vi "Check Dependencies with Preview.vi"(8 "error in (no error)":errorcluster, 11 "Builder in":refnum<class "Builder.lvclass">) -> (0 "error out":errorcluster, 3 "Builder out":refnum<class "Builder.lvclass">)   [LabVIEW 2019, in "Builder.lvclass"]
uses:
  Builder.lvclass
  Builder.lvclass/Builder.ctl
  <vilib>/Utility/lvfile.llb/LVFileType.ctl
  <vilib>/AppBuilder/AB_API/PPL/NI_AB_API_PPL.lvclass
  <vilib>/Utility/lvfile.llb/NI_FileType.lvlib
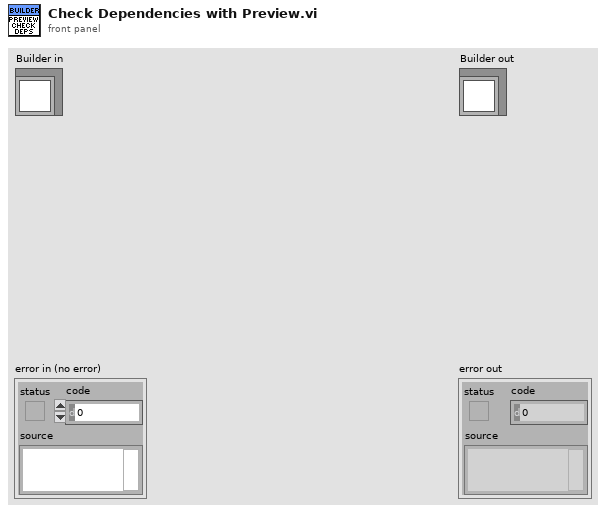
[diagram p1: front panel]
types:
  T1 = typedef "NI_FileType.lvlib/LVFileType.ctl" = enum32{"Invalid file", "Unknown type", "Instrument", "Control", "Polymorphic VI", "Project", "Library", "LVClass", "XControl", "XNode", "Shared library", ".NET assembly", "ActiveX interface", "CIN", "Run-time menu", "Palette menu", "Help file", "LLB", "XNode Edit Dependency", "Class Private Data Control", "Statechart", "MathScript .m file", "Ladder Diagram", "LVLibp", "XNode Build Dependency"}
  T2 = typedef "AB_Dependency.ctl" = cluster{"path":path, "delimited name":string, "type":T1}
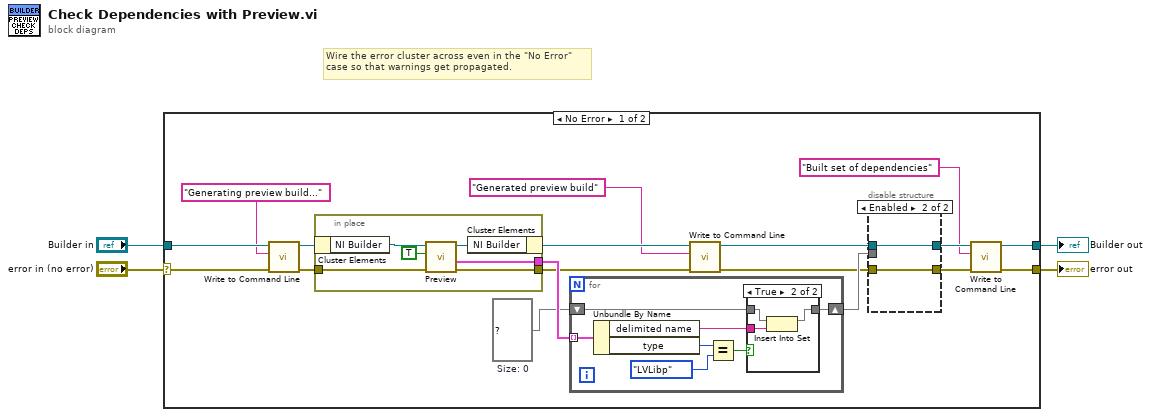
[diagram p0: block diagram]
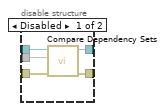
[diagram p2: hidden frame]
diagram:
  # "Wire the error cluster across even in the \"No Error\"\ncase so that warnings get propagated."
  n1 = case shown="No Error" "error in (no error)" {
    selector: "error in (no error)" -> [w22 w48]
    tunnel: [w10 w48] -> w3
    tunnel: [w8 w47] -> w1
    tunnel: "Builder in" -> [w15 w47]
    frame No Error {
      w20 = set{string} {}  # Size: 0
      n2 = call "Write to Command Line.vi"("error in (no error)"=w22, "Message"="Generating preview build...", "Builder in"=w15) -> ("error out"=w16:errorcluster, "Builder out"=w14:refnum<class "Builder.lvclass">)  [unwired: 7 in]
      n3 = in-place {
        in-place-border: w16 -> [w43]
        in-place-border: [w42] -> w18
        in-place-border: [w41] -> w21
        n4 = in-place-cluster #1(w14) -> ("NI Builder"=w46:refnum<class "NI_AB_API_PPL.lvclass">)
        n5 = call-dynamic "Preview.vi"("error in (no error)"=w43, "collect dependencies? (F)"=TRUE, "PPL in"=w46) -> ("error out"=w42:errorcluster, "Dependencies"=w41:T2[], "PPL out"=w45:refnum<class "NI_AB_API_PPL.lvclass">)  [unwired: 5 in, 1 out]
        n6 = in-place-cluster #1("NI Builder"=w45) -> (w12:refnum<class "Builder.lvclass">)
      }
      n7 = for {
        tunnel: w21 -> [w36] mode=indexing
        shift-right: [w31] -> w19
        shift-left: w20 -> [w30]
        n8 = Unbundle By Name(w36) -> ("delimited name"=w33:string, "type"=w35:T1)
        n9 = Equal?(x=w35, y=LVFileType."LVLibp") -> (x = y?=w32:bool)
        n10 = case shown="True" w32 {
          tunnel: w33 -> [_ w40]
          tunnel: [w37 w39] -> w31
          tunnel: w30 -> [w37 w38]
          frame False {
          }
          frame True {
            n11 = Insert Into Set(10:w40, 11:w38) -> (3:w39:set{string})  [unwired: 1 out]
          }
        }
      }
      n12 = call "Write to Command Line.vi"("error in (no error)"=w18, "Message"="Generated preview build", "Builder in"=w12) -> ("error out"=w13:errorcluster, "Builder out"=w11:refnum<class "Builder.lvclass">)  [unwired: 7 in]
      n13 = disable-structure shown="Enabled" {
        disable-tunnel: w19 -> [w27 _]
        disable-tunnel: w13 -> [w26 w28]
        disable-tunnel: [w25 w28] -> w17
        disable-tunnel: w11 -> [w24 w29]
        disable-tunnel: [w23 w29] -> w9
        frame Disabled {
          n14 = call "Compare Dependency Sets.vi"("error in (no error)"=w26, "Scanned"=w27, "Builder in"=w24) -> ("error out"=w25:errorcluster, "Builder out"=w23:refnum<class "Builder.lvclass">)  [unwired: 7 in]
        }
        frame Enabled {
        }
      }
      n15 = call "Write to Command Line.vi"("error in (no error)"=w17, "Message"="Built set of dependencies", "Builder in"=w9) -> ("error out"=w10:errorcluster, "Builder out"=w8:refnum<class "Builder.lvclass">)  [unwired: 7 in]
    }
    frame Error {
    }
  }
  "error out" <- w3
  "Builder out" <- w1
